vi "Параметры мишени в строку (SubVI).vi"(2 "Кластер параметров мишени":T1) -> (0 "Параметры мишени строка":string)   [LabVIEW 2013]
doc: "Преобразует параметры мишени в строку для дальнейшей записи в файл"
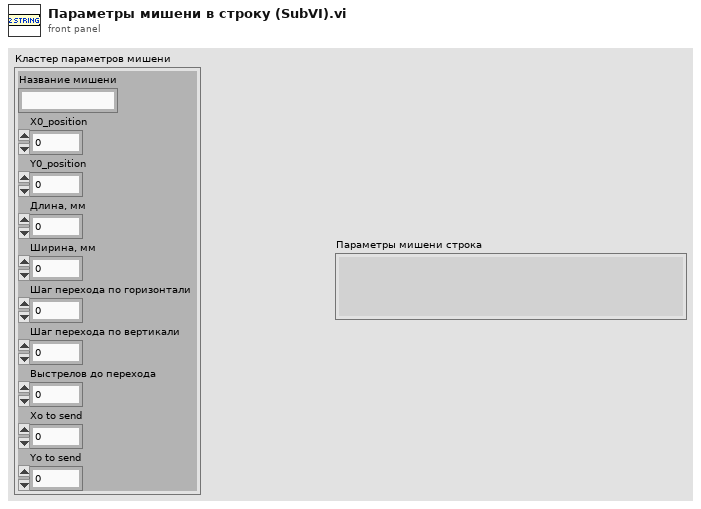
[diagram p1: front panel]
types:
  T1 = cluster{"Название мишени":string, "Х0_position":u16, "Y0_position":u16, "Длина, мм":u16, "Ширина, мм":u16, "Шаг перехода по горизонтали":dbl, "Шаг перехода по вертикали":dbl, "Выстрелов до перехода":u16, "Xo to send ":u16, "Yo to send":u16}
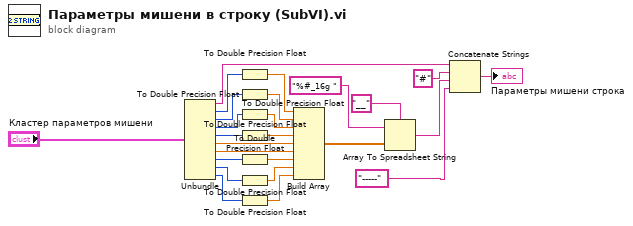
[diagram p0: block diagram]
diagram:
  n1 = Unbundle("Кластер параметров мишени") -> ("Название мишени"=w12:string, "Х0_position"=w4:u16, "Y0_position"=w14:u16, "Длина, мм"=w15:u16, "Ширина, мм"=w16:u16, "Шаг перехода по горизонтали"=w5:dbl, "Шаг перехода по вертикали"=w6:dbl, "Выстрелов до перехода"=w23:u16, "Xo to send"=w24:u16, "Yo to send"=w25:u16)
  n2 = To Double Precision Float(number=w4) -> (double precision float=w13:dbl)
  n3 = To Double Precision Float(number=w14) -> (double precision float=w19:dbl)
  n4 = To Double Precision Float(number=w15) -> (double precision float=w18:dbl)
  n5 = To Double Precision Float(number=w16) -> (double precision float=w17:dbl)
  n6 = To Double Precision Float(number=w23) -> (double precision float=w20:dbl)
  n7 = To Double Precision Float(number=w24) -> (double precision float=w21:dbl)
  n8 = To Double Precision Float(number=w25) -> (double precision float=w22:dbl)
  n9 = Build Array(w13, w19, w18, w17, w5, w6, w20, w21, w22) -> (w9:dbl[])
  n10 = Array To Spreadsheet String(delimiter (Tab)="__", array=w9, 3:"%#_16g " ("format string")) -> (spreadsheet string=w11:string)
  n11 = Concatenate Strings(w12, "#" ("delimiter (Tab)"), w11, "-----" ("string")) -> (→"Параметры мишени строка":string)
